vi "DriveTuningPathGenerator.vi"() -> (4 "Left Drive Motion Profile":T2[](array[typedef]), 6 "Right Drive Motion Profile":T2[](array[typedef]), 8 "Go":bool)   [LabVIEW 2017]
uses:
  General/MotionProfiling/TypeDefs/MotionProfileGeneratorParams.ctl
  <vilib>/Rock Robotics/WPI/ThirdParty/Phoenix-LabVIEW/Motor Controller/Controls/CTRE_Phoenix_MotorControl_TrajectoryPointTimeDur.ctl
  Pathfinder/Pathfinder-LabVIEW/Pathfinder-Lib/VIs/Segment.ctl
  ArgosLib/Signal Processing/TypeDefs/EdgeDetector_Type.ctl
  ArgosLib/ArgosLib.lvlib
  Pathfinder/Pathfinder-LabVIEW/Pathfinder-Lib/Pathfinder.lvlib
panel:
  out "Right Drive Motion Profile Graph":T1(graph)
  out "Left Drive Motion Profile Graph":T1(graph)
  in  "MotionProfileGeneratorParameters":T3={"Trajectory Point Interval (ms)"=10, "Maximum Travel Speed (units/s)"=500.0, "Velocity Ramp Time (ms)"=400.0, "Acceleration Ramp Time (ms)"=200.0} {"Acceleration Ramp Time (ms)" min=1.0; "Velocity Ramp Time (ms)" min=1.0; "Maximum Travel Speed (units/s)" min=0.0; "Trajectory Point Interval (ms)" items=["TrajectoryDuration_0ms"=0, "TrajectoryDuration_5ms"=5, "TrajectoryDuration_10ms"=10, "TrajectoryDuration_20ms"=20, "TrajectoryDuration_30ms"=30, "TrajectoryDuration_40ms"=40, "TrajectoryDuration_50ms"=50, "TrajectoryDuration_100ms"=100]}
  in  "Reverse Direction":bool
  in  "Send Motion Profiles":bool
  in  "End Dist":dbl
  in  "Start Dist":dbl
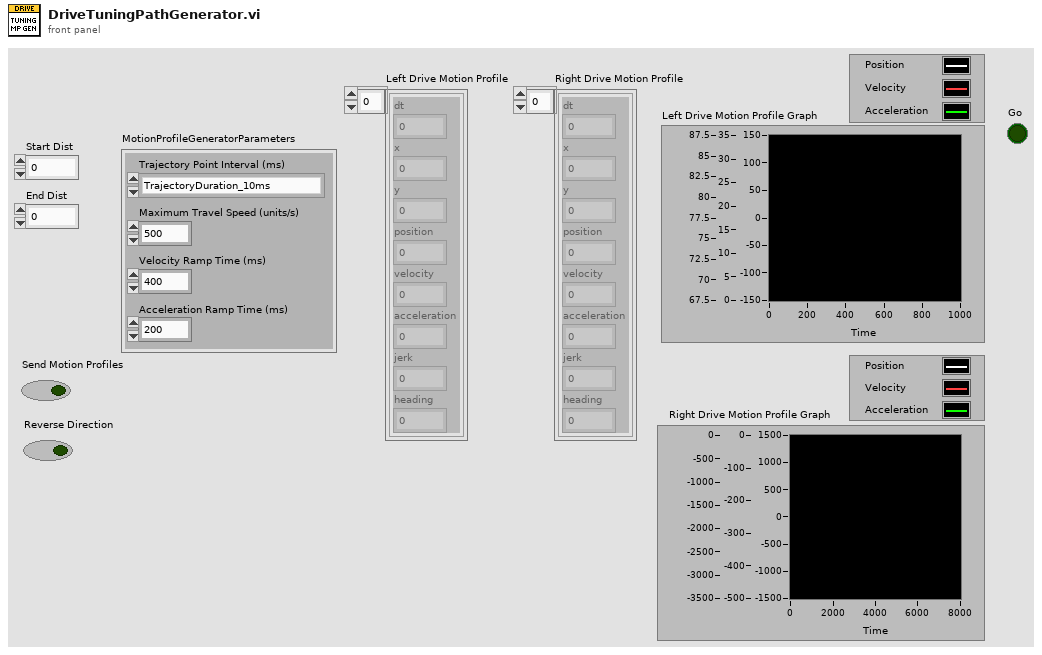
[diagram p1: front panel]
types:
  T1 = cluster{dbl, "Trajectory Point Interval (ms)":i32, dbl[][]}
  T2 = typedef "Pathfinder.lvlib/Segment.ctl" = cluster{"dt":dbl, "x":dbl, "y":dbl, "position":dbl, "velocity":dbl, "acceleration":dbl, "jerk":dbl, "heading":dbl}
  T3 = typedef "MotionProfileGeneratorParams.ctl" = cluster{"Trajectory Point Interval (ms)":T4, "Maximum Travel Speed (units/s)":dbl, "Velocity Ramp Time (ms)":dbl, "Acceleration Ramp Time (ms)":dbl}
  T4 = typedef "CTRE_Phoenix_MotorControl_TrajectoryPointTimeDur.ctl" = i32
  T5 = typedef "ArgosLib.lvlib/EdgeDetector_Type.ctl" = enum16{"RisingEdge", "FallingEdge", "Both"}
  T6 = typedef "TrajectoryPoint.ctl" = cluster{"Position ":dbl, "Velocity ":dbl, "Time (ms)":T4, "Last Point":bool}
  T7 = cluster{dbl, "Trajectory Point Interval (ms)":T4, dbl[][]}
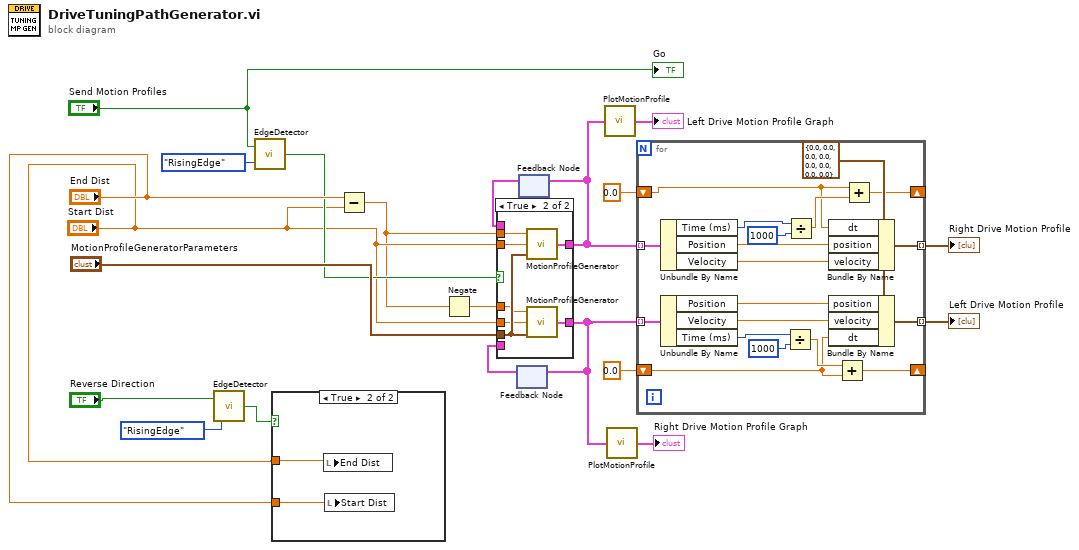
[diagram p0: block diagram]
diagram:
  n1 = call "EdgeDetector.vi"("DetectorType"=EdgeDetector_Type."RisingEdge", "Input"="Reverse Direction") -> ("Edge"=w17:bool)
  n2 = call "EdgeDetector.vi"("DetectorType"=EdgeDetector_Type."RisingEdge", "Input"="Send Motion Profiles") -> ("Edge"=w12:bool)
  n3 = case shown="True" w17 {
    tunnel: "End Dist" -> [_ w23]
    tunnel: "Start Dist" -> [_ w22]
    frame False {
    }
    frame True {
      n4 = local write "End Dist"(w22) -> ()
      n5 = local write "Start Dist"(w23) -> ()
    }
  }
  n6 = Subtract(x="End Dist", y="Start Dist") -> (x-y=w8:dbl)
  n7 = Negate(x=w8) -> (-x=w7:dbl)
  n8 = feedback #1() -> (w14:T6[])  [unwired: 1 in]
  n9 = feedback #2() -> (w13:T6[])  [unwired: 1 in]
  n10 = case shown="True" w12 {
    tunnel: w8 -> [_ w32]
    tunnel: "MotionProfileGeneratorParameters" -> [_ w31]
    tunnel: "Start Dist" -> [_ w30]
    tunnel: [w24 w29] -> w6
    tunnel: [w25 w28] -> w5
    tunnel: w14 -> [w25 _]
    tunnel: w13 -> [w24 _]
    tunnel: "Start Dist" -> [_ w27]
    tunnel: w7 -> [_ w26]
    frame False {
    }
    frame True {
      n11 = call "MotionProfileGenerator.vi"("MotionProfileGeneratorParameters"=w31, "Starting Position (units)"=w30, "Travel Distance (units)"=w32) -> ("Trajectory Points"=w29:T6[])
      n12 = call "MotionProfileGenerator.vi"("MotionProfileGeneratorParameters"=w31, "Starting Position (units)"=w27, "Travel Distance (units)"=w26) -> ("Trajectory Points"=w28:T6[])
    }
  }
  n13 = feedback-in #1(w5) -> ()
  n14 = feedback-in #2(w6) -> ()
  n15 = call "PlotMotionProfile.vi"("Trajectory Points"=w6) -> ("MotionProfileGraph"=→"Left Drive Motion Profile Graph":T7)
  n16 = call "PlotMotionProfile.vi"("Trajectory Points"=w5) -> ("MotionProfileGraph"=→"Right Drive Motion Profile Graph":T7)
  n17 = for {
    tunnel: w6 -> [w51] mode=indexing
    tunnel: w5 -> [w50] mode=indexing
    tunnel: [w47] -> w2 mode=indexing
    tunnel: [w43] -> w1 mode=indexing
    shift-right: [w38] -> _
    shift-left: 0.0 -> [w36]
    shift-right: [w35] -> _
    shift-left: 0.0 -> [w33]
    w45 = T2 {"dt"=0.0, "x"=0.0, "y"=0.0, "position"=0.0, "velocity"=0.0, "acceleration"=0.0, "jerk"=0.0, "heading"=0.0} ("trajectory point")
    n18 = Unbundle By Name(w51) -> ("Time (ms)"=w39:T4, "Position"=w49:dbl, "Velocity"=w48:dbl)
    n19 = Unbundle By Name(w50) -> ("Position"=w44:dbl, "Velocity"=w42:dbl, "Time (ms)"=w41:T4)
    n20 = Divide(x=w41, y=1000) -> (x/y=w37:dbl)
    n21 = Divide(x=w39, y=1000) -> (x/y=w34:dbl)
    n22 = Bundle By Name(cluster=w45, "dt"=w33, "position"=w49, "velocity"=w48) -> (w47:T2)
    n23 = Bundle By Name(cluster=w45, "position"=w44, "velocity"=w42, "dt"=w36) -> (w43:T2)
    n24 = Add(x=w37, y=w36) -> (x+y=w38:dbl)
    n25 = Add(x=w33, y=w34) -> (x+y=w35:dbl)
  }
  "Right Drive Motion Profile" <- w2
  "Left Drive Motion Profile" <- w1
  "Go" <- "Send Motion Profiles"
